vi "Inspect Submission.vi"(8 "error in (no error)":errorcluster, 11 "Folder":path) -> (0 "error out":errorcluster, 2 "Inspection Result":string, 3 "Result":bool)   [LabVIEW 2024, in "Word Search Scorer.lvlib"]
uses:
  Word Search Scorer.lvlib
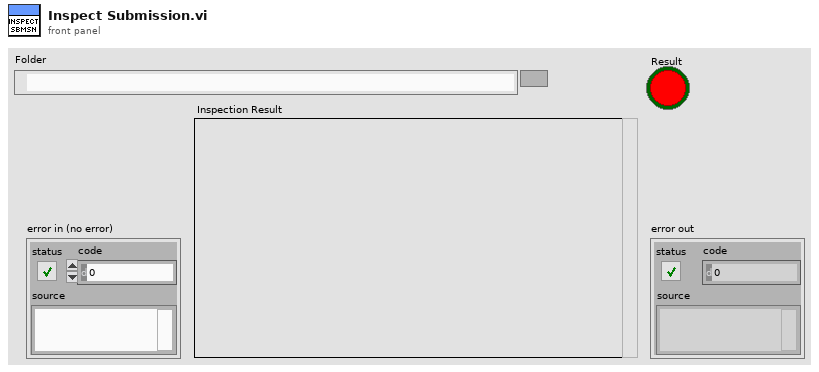
[diagram p1: front panel]
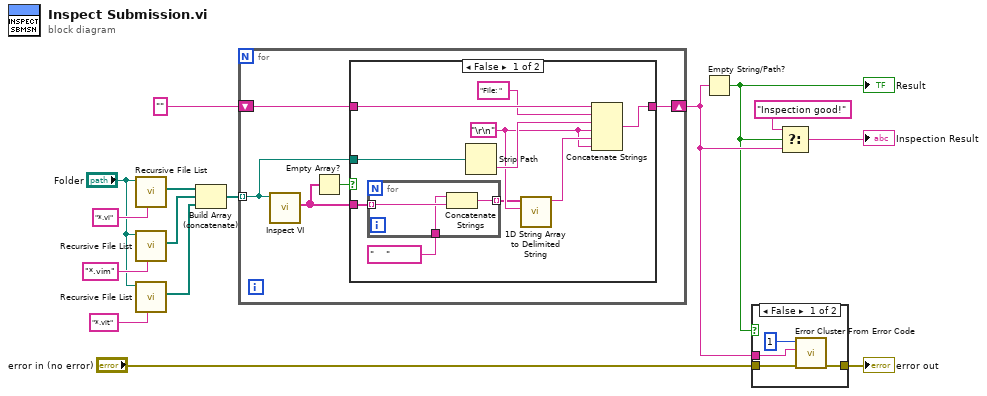
[diagram p0: block diagram]
diagram:
  n1 = call <vilib>:"Recursive File List.vi"("pattern"="*.vi", "Folder Path"="Folder") -> ("All Files in Dir"=w11:path[])  [unwired: 5 in, 4 out]
  n2 = call <vilib>:"Recursive File List.vi"("pattern"="*.vim", "Folder Path"="Folder") -> ("All Files in Dir"=w10:path[])  [unwired: 5 in, 4 out]
  n3 = call <vilib>:"Recursive File List.vi"("pattern"="*.vit", "Folder Path"="Folder") -> ("All Files in Dir"=w9:path[])  [unwired: 5 in, 4 out]
  n4 = Build Array (concatenate)(w11, w10, w9) -> (w8:path[])
  n5 = for {
    tunnel: w8 -> [w17] mode=indexing
    shift-right: [w16] -> w2
    shift-left: "" -> [w20]
    n6 = call "Inspect VI.vi"("VI Path"=w17) -> ("Issues"=w19:string[])  [unwired: 9 in, 1 out]
    n7 = Empty Array?(array=w19) -> (empty?=w18:bool)
    n8 = case shown="False" w18 {
      tunnel: w20 -> [w30 w34]
      tunnel: w19 -> [w23 _]
      tunnel: w17 -> [w28 _]
      tunnel: [w24 w34] -> w16
      frame False {
        w25 = "\r\n"
        n9 = for {
          tunnel: w23 -> [w33] mode=indexing
          tunnel: "    " -> [w32]
          tunnel: [w31] -> w21 mode=indexing
          n10 = Concatenate Strings(w32, w33) -> (w31:string)
        }
        n11 = Strip Path(path=w28) -> (name=w27:string)  [unwired: 1 out]
        n12 = call <vilib>:"1D String Array to Delimited String.vi"("delimiter"=w25, "string array"=w21) -> ("delimited string"=w26:string)  [unwired: 9 in]
        n13 = Concatenate Strings(w30, "File: " ("string"), w27, w25, w26, w25) -> (w24:string)
      }
      frame True {
      }
    }
  }
  n14 = Empty String/Path?(string/path=w2) -> (empty?=w1:bool)
  "Result" <- w1
  n15 = case shown="False" w1 {
    tunnel: "error in (no error)" -> [w38 w39]
    tunnel: [w37 w39] -> w3
    tunnel: w2 -> [w35 _]
    frame False {
      n16 = call <vilib>:"Error Cluster From Error Code.vi"("error in (no error)"=w38, "error message (\"\")"=w35, "error code (0)"=1) -> ("error out"=w37:errorcluster)  [unwired: 6 in]
    }
    frame True {
    }
  }
  "error out" <- w3
  n17 = Select(t="Inspection good!", s=w1, f=w2) -> (s? t:f=→"Inspection Result":string)
